vi "Dot number to bytes.vi"(10 "Hex String":bool, 11 "Dot # (Decimal String)":string) -> (0 "4th Byte":u8, 1 "3rd Byte":u8, 2 "2nd Byte":u8, 3 "1st Byte (MSB)":u8, 4 "5th Byte":u8, 5 "Byte Array":u8[](array[numeric]), 6 "6th Byte":u8)   [LabVIEW 2020]
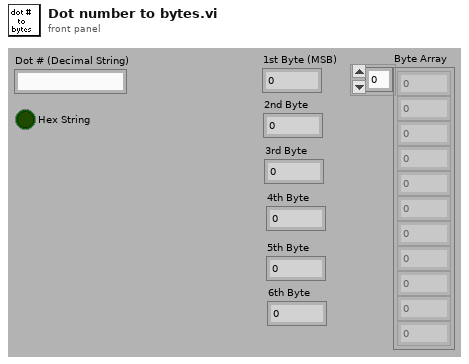
[diagram p1: front panel]
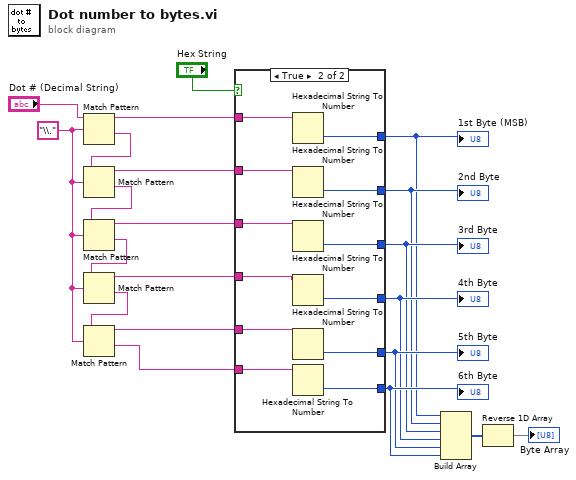
[diagram p0: block diagram]
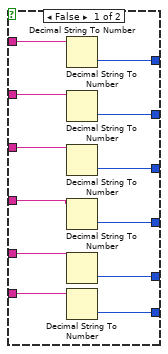
[diagram p2: hidden frame]
diagram:
  w21 = "\\." ("regular expression")
  n1 = Match Pattern(string="Dot # (Decimal String)", regular expression=w21) -> (before substring=w15:string, after substring=w19:string)  [unwired: 1 in, 2 out]
  n2 = Match Pattern(string=w19, regular expression=w21) -> (before substring=w14:string, after substring=w18:string)  [unwired: 1 in, 2 out]
  n3 = Match Pattern(string=w18, regular expression=w21) -> (before substring=w13:string, after substring=w17:string)  [unwired: 1 in, 2 out]
  n4 = Match Pattern(string=w17, regular expression=w21) -> (before substring=w12:string, after substring=w16:string)  [unwired: 1 in, 2 out]
  n5 = Match Pattern(string=w16, regular expression=w21) -> (before substring=w11:string, after substring=w10:string)  [unwired: 1 in, 2 out]
  n6 = case shown="True" "Hex String" {
    tunnel: w15 -> [w33 w45]
    tunnel: w14 -> [w32 w44]
    tunnel: w13 -> [w31 w43]
    tunnel: w12 -> [w30 w42]
    tunnel: w11 -> [w29 w41]
    tunnel: w10 -> [w28 w40]
    tunnel: [w27 w39] -> w3
    tunnel: [w26 w38] -> w4
    tunnel: [w25 w37] -> w5
    tunnel: [w24 w36] -> w6
    tunnel: [w23 w35] -> w7
    tunnel: [w22 w34] -> w8
    frame False {
      n7 = Decimal String To Number(string=w33) -> (number=w27:i32)  [unwired: 2 in, 1 out]
      n8 = Decimal String To Number(string=w32) -> (number=w26:i32)  [unwired: 2 in, 1 out]
      n9 = Decimal String To Number(string=w31) -> (number=w25:i32)  [unwired: 2 in, 1 out]
      n10 = Decimal String To Number(string=w30) -> (number=w24:i32)  [unwired: 2 in, 1 out]
      n11 = Decimal String To Number(string=w29) -> (number=w23:i32)  [unwired: 2 in, 1 out]
      n12 = Decimal String To Number(string=w28) -> (number=w22:i32)  [unwired: 2 in, 1 out]
    }
    frame True {
      n13 = Hexadecimal String To Number(string=w45) -> (number=w39:u32)  [unwired: 2 in, 1 out]
      n14 = Hexadecimal String To Number(string=w44) -> (number=w38:u32)  [unwired: 2 in, 1 out]
      n15 = Hexadecimal String To Number(string=w43) -> (number=w37:u32)  [unwired: 2 in, 1 out]
      n16 = Hexadecimal String To Number(string=w42) -> (number=w36:u32)  [unwired: 2 in, 1 out]
      n17 = Hexadecimal String To Number(string=w41) -> (number=w35:u32)  [unwired: 2 in, 1 out]
      n18 = Hexadecimal String To Number(string=w40) -> (number=w34:u32)  [unwired: 2 in, 1 out]
    }
  }
  "1st Byte (MSB)" <- w3
  "2nd Byte" <- w4
  "3rd Byte" <- w5
  "4th Byte" <- w6
  "5th Byte" <- w7
  "6th Byte" <- w8
  n19 = Build Array(w3, w4, w5, w6, w7, w8) -> (w2:u32[])
  n20 = Reverse 1D Array(array=w2) -> (reversed array=→"Byte Array":u32[])
